vi "Close Display.vi"(8 "error in (no error)":errorcluster, 11 "Report Viewer in":refnum<class "Report Viewer.lvclass">) -> (0 "error out":errorcluster, 3 "Report Viewer out":refnum<class "Report Viewer.lvclass">)   [LabVIEW 2019, in "Report Viewer.lvlib" / "Report Viewer.lvclass"]
uses:
  Library/Report Viewer.lvclass
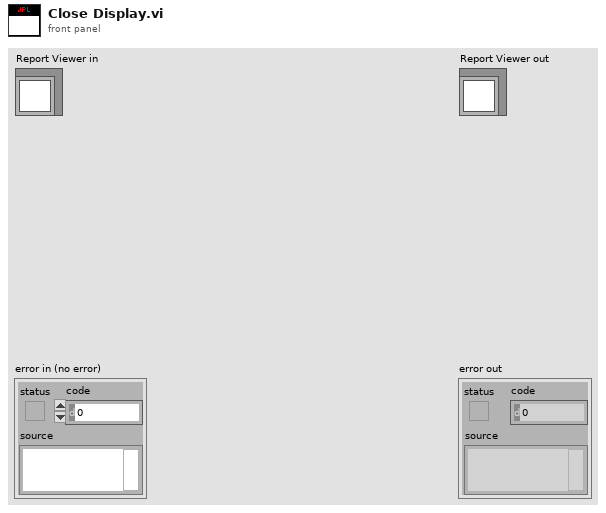
[diagram p1: front panel]
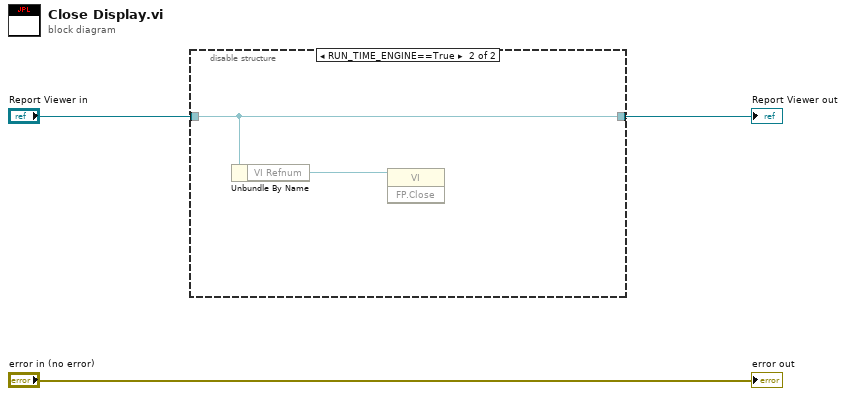
[diagram p0: block diagram]
diagram:
  n1 = disable-structure shown="RUN_TIME_ENGINE==True" {
    disable-tunnel: "Report Viewer in" -> [w4 w6]
    disable-tunnel: [w4 w6] -> w1
    frame condition #0 (active) {
    }
    frame condition #1 {
      n2 = Unbundle By Name(w6) -> ("VI Refnum"=w5:refnum<vi>)
      n3 = invoke class="VI" method="FP.Close"(reference=w5) -> ()  [unwired: 2 in, 3 out]
    }
  }
  "Report Viewer out" <- w1
  "error out" <- "error in (no error)"
